vi "SLL DE AI Circular Buffer.vi"(6 "Pointers":T3=enum."Pointer 4", 7 "Options":T4=enum."Write", 8 "error in (no error)":errorcluster, 9 "Time In":timestamp[](array[timestamp]), 11 "Input Data":sgl[][](array[numeric])) -> (0 "error Out":errorcluster, 1 "Data Overflow?":T1, 2 "Output points":sgl[](array[numeric]), 3 "Output Data":sgl[][](array[numeric]), 4 "Multi Time Stamp":timestamp[](array[timestamp]), 5 "Single Time Stamp":timestamp)   [LabVIEW 2009]
doc: "This vi acts as a circular buffer for Analog input channel data storage. \nOutput Array- Column coresponds to single channel data.\nSingle Point data of all channels will avilable, When 'Data Point' case will executes.\nYou can get continous data in two mode 'Read Pointer 1' and 'Read Pointer 2'.\nInitializing Pointer is recommeded to avoid overflow\n\nCreated by Yogesh Redemptor, \nCopyright © 2009, Soliton Technologies.\nAll rights reserved."
uses:
  Controls/SLL DE Circular Buffer Options.ctl
  Controls/SLL DE Circular Buffer Pointers List.ctl
  Controls/SLL DE List of Analog Inputs.ctl
  Controls/SLL DE Circular Buffer Overflow Info.ctl
  Controls/SLL DE DAQ Parameters LV2Global Options.ctl
panel:
  in  "List of Analog Inputs":T2
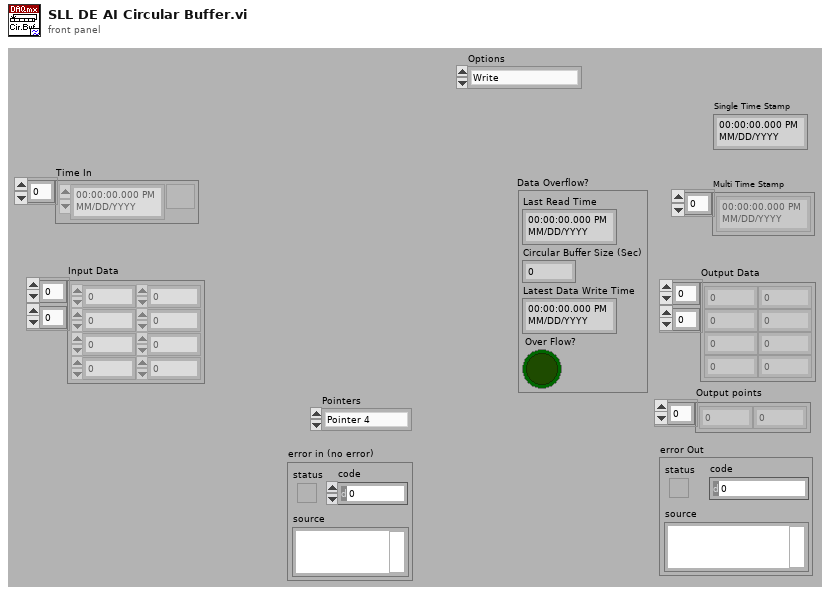
[diagram p1: front panel]
types:
  T1 = typedef "SLL DE Circular Buffer Overflow Info.ctl" = cluster{"Last Read Time":timestamp, "Circular Buffer Size (Sec)":dbl, "Latest Data Write Time":timestamp, "Over Flow?":bool}
  T2 = typedef "SLL DE List of Analog Inputs.ctl" = enum16{"None"}
  T3 = typedef "SLL DE Circular Buffer Pointers List.ctl" = enum16{"Graph Pointer", "File Log Pointer", "Pointer 3", "Pointer 4"}
  T4 = typedef "SLL DE Circular Buffer Options.ctl" = enum16{"Initialize", "Init Pointer X", "Write", "Read Single Value", "Read Pointer X (Multi Value)", "Clear Data"}
  T5 = typedef "SLL DE DAQ Parameters LV2Global Options.ctl" = enum16{"Read", "Write"}
  T6 = cluster{"Buffer Length":i32, "Write Pointer":i32, "Write Time":timestamp}
  T7 = cluster{"Read Pointer X Pointer":i32, "Pointer X Overflow?":bool, "Read Pointer X Time":timestamp}
  T8 = typedef "SLL DE DAQ Engine Parameters.ctl" = cluster{"Enable Engines":cluster{"AI Enable":bool, "AO Enable":bool, "DI Enable":bool, "DO Enable":bool}, "DAQ Control Type":cluster{"Analog Input":enum16{"Finite", "Continuous", "Driver"}, "Analog Output":enum16{"Finite", "Continuous", "Driver"}, "Digital Input":enum16{"Finite", "Continuous", "Driver"}, "Digital Output":enum16{"Finite", "Continuous", "Driver"}}, "DAQ Parameters":cluster{"AI Sampling Rate (Samples/Sec)":dbl, "MvgAVG Window Size (# of Points)":i32, "Enable Filter":bool, "Enable MvgAVG":bool, "Circular Buffer Size (Sec)":dbl, "AO Sampling Rate (Samples/Sec)":dbl, "Graph Update Rate (Samples/Sec)":dbl, "File Logging Rate (Samples/Sec)":i32}, "AO Safe Values":cluster{"Analog Outputs Name":T9, "Analog Outputs Safe Value":dbl}[], "DO Safe Values":cluster{"Digital Outputs Name":T10, "Digital Outputs Safe Value":bool}[], "DO Interconnected Lines":cluster{"First DO Line":string, "Second DO Line":string}[], "AI Channels Unit":cluster{"Channel Name":T2, "Channel Type":T11}[], "Units Information":cluster{"Channel Type":T11, "Unit Text":string, "Maximum":dbl, "Minmum":dbl, "Increments":dbl}[]}
  T9 = typedef "SLL DE List of Analog Outputs.ctl" = enum16{"None"}
  T10 = typedef "SLL DE List of Digital Outputs.ctl" = enum16{"STATION1_START TEST", "STATION1_STOP TEST", "STATION1_LIGHT1", "STATION1_LIGHT2", "STATION1_LIGHT3", "STATION2_START TEST", "STATION2_STOP TEST", "STATION2_LIGHT1", "STATION2_LIGHT2", "STATION2_LIGHT3", "STATION3_START TEST", "STATION3_STOP TEST", "STATION3_LIGHT1", "STATION3_LIGHT2", "STATION3_LIGHT3", "STATION4_START TEST", "STATION4_STOP TEST", "STATION4_LIGHT1", "STATION4_LIGHT2", "STATION4_LIGHT3"}
  T11 = typedef "SLL DE List of AI Channel Type.ctl" = enum16{"Pressure", "Flow", "Temperature", "Time Scale", "Voltage", "Current", "Frequency", "Sound", "Speed", "Torque", "Distance", "Channel Type 1", "Channel Type 2", "Channel Type 3"}
  T12 = cluster{"Read Pointer X Pointer":i32, "Pointer X Overflow?":bool, "Read Pointer X Time":timestamp}[]
  T13 = cluster{"Read Pointer X Time":timestamp, "Circular Buffer Size (Sec)":dbl, "Write Time":timestamp, bool}
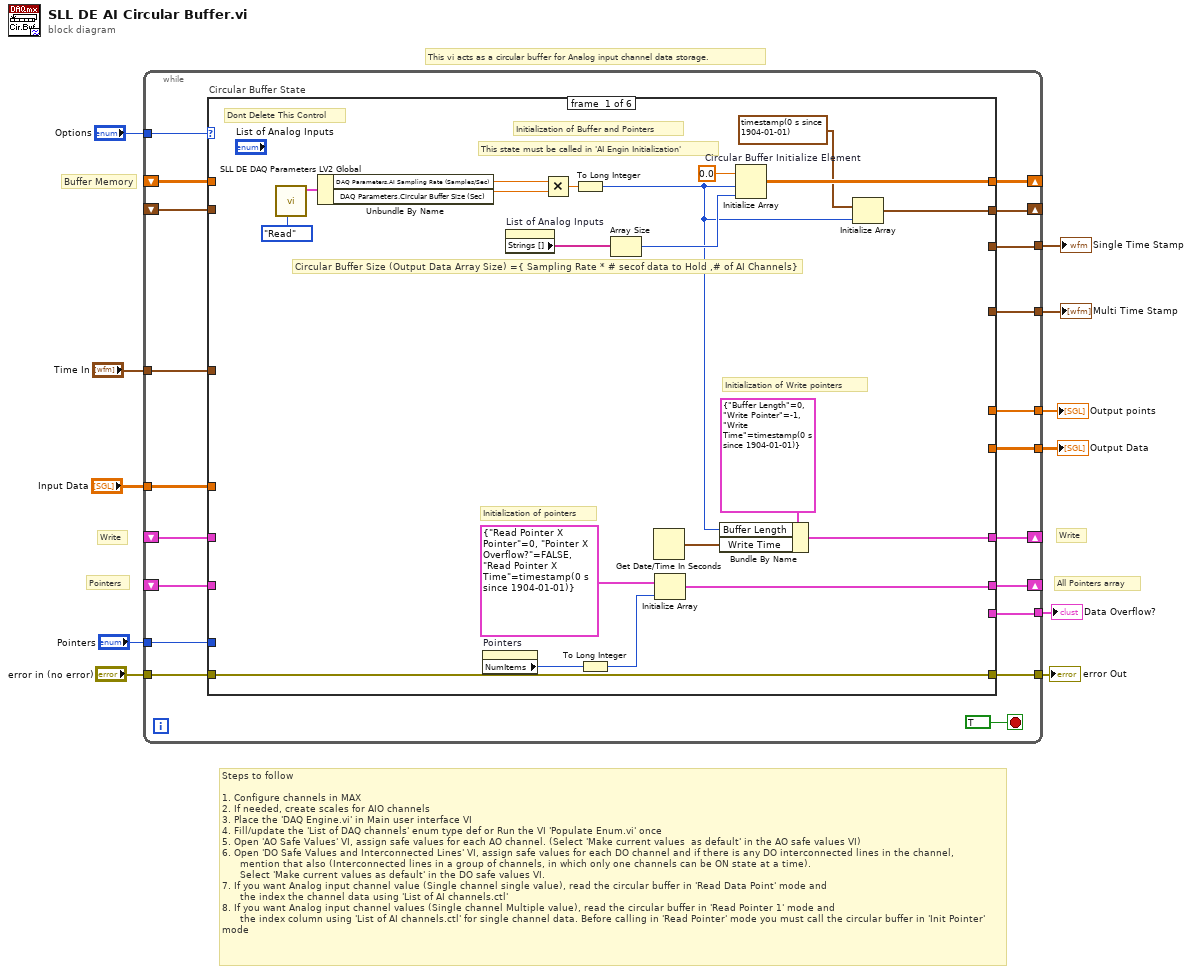
[diagram p0: block diagram]
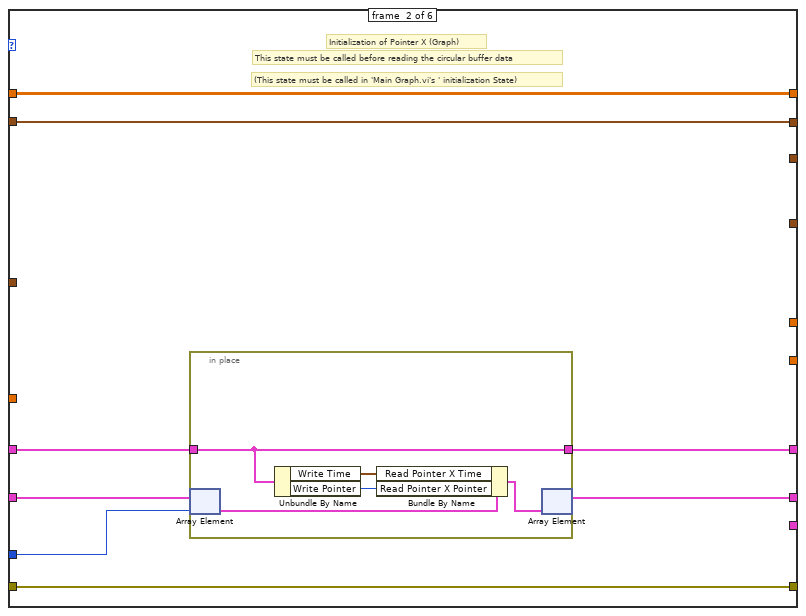
[diagram p2: hidden frame]
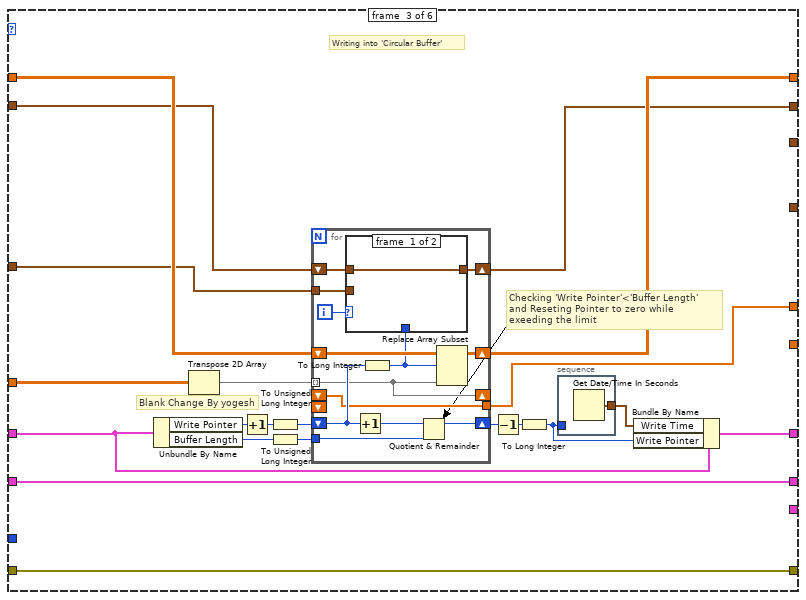
[diagram p3: hidden frame]
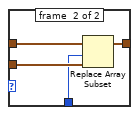
[diagram p4: hidden frame]
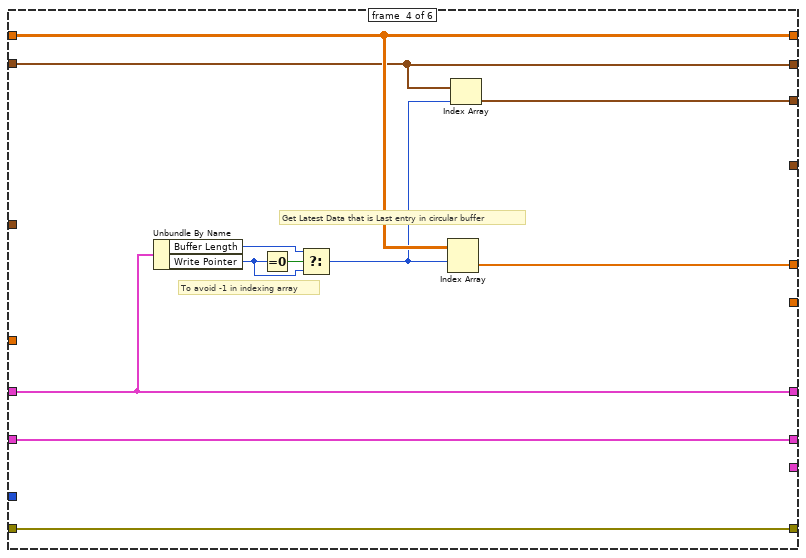
[diagram p5: hidden frame]
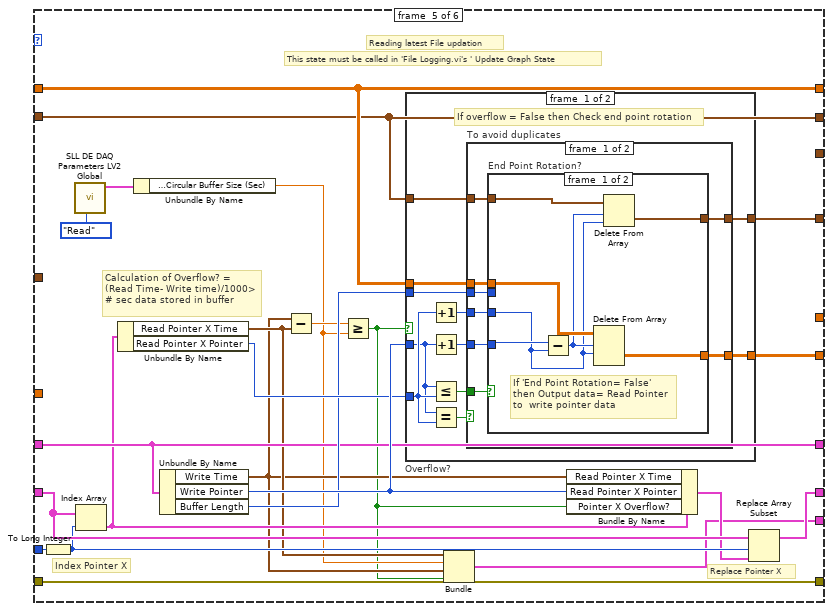
[diagram p6: hidden frame]
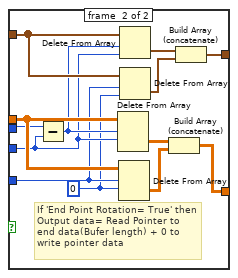
[diagram p7: hidden frame]
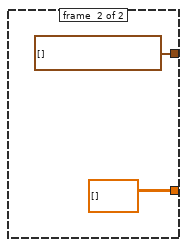
[diagram p8: hidden frame]
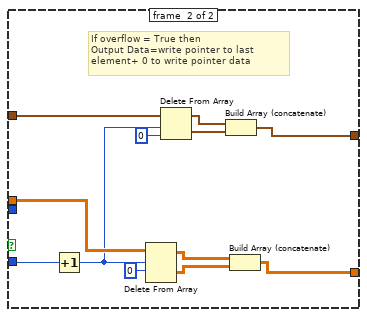
[diagram p9: hidden frame]
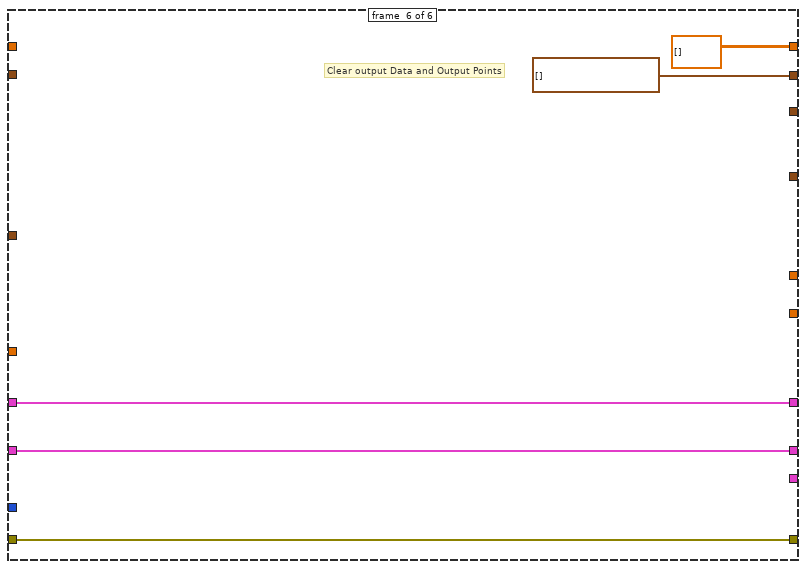
[diagram p10: hidden frame]
diagram:
  # "Steps to follow\n\n1.\tConfigure channels in MAX\n2.\tIf needed, create scales for AIO channels\n3.\tPlace the 'DAQ Engine.vi' in Main user interface VI\n4.\tFill/update the 'List of DAQ channels' enum type def or Run the VI 'Populate Enum.vi' once\n5.\tOpen 'AO Safe Values' VI, assign safe values for each AO channel. (Select 'Make current values  as default' in the AO safe values VI)\n6.\tOpen 'DO Safe Values and Interconnected Lines' VI, assign safe values for each DO channel and if there is any DO interconnected lines in the channel,\n      mention that also (Interconnected lines in a group of channels, in which only one channels can be ON state at a time). \n      Select 'Make current values as default' in the DO safe values VI.\n7.\tIf you want Analog input channel value (Single channel single value), read the circular buffer in 'Read Data Point' mode and \n      the index the channel data using 'List of AI channels.ctl' \n8.\tIf you want Analog input channel values (Single channel Multiple value), read the circular buffer in 'Read Pointer 1' mode and \n      the index column using 'List of AI channels.ctl' for single channel data. Before calling in 'Read Pointer' mode you must call the circular buffer in 'Init Pointer' mode"
  # "Buffer Memory"
  # "Write"
  # "Write"
  # "Pointers"
  # "All Pointers array"
  # "This vi acts as a circular buffer for Analog input channel data storage."
  n1 = while {
    tunnel: "Options" -> [w31]
    shift-right: [w29] -> _
    shift-left: _ -> [w27]
    shift-right: [w28] -> _
    shift-left: _ -> [w26]
    tunnel: "Input Data" -> [w25]
    tunnel: [w24] -> w10
    shift-right: [w23] -> _
    shift-left: _ -> [w22]
    tunnel: [w21] -> w9
    tunnel: "error in (no error)" -> [w20]
    tunnel: [w19] -> w7
    tunnel: "Pointers" -> [w18]
    tunnel: "Time In" -> [w17]
    shift-right: [w16] -> _
    shift-left: _ -> [w15]
    tunnel: [w14] -> w3
    tunnel: [w13] -> w2
    tunnel: [w12] -> w1
    stop <- TRUE stop-if-true
    n2 = case "Circular Buffer State" shown="\"Read Pointer X (Multi Value)\"" w31 {
      tunnel: [w51 w59 w81 w114 w138 sgl[][] []] -> w29
      tunnel: [w46 w55 w85 w115 w127 w196] -> w28
      tunnel: w27 -> [_ w59 w83 w114 w138 _]
      tunnel: w26 -> [_ w57 w85 w115 w130 w196]
      tunnel: w25 -> [_ _ w84 _ _ _]
      tunnel: [_ _ w69 w113 _ _] -> w24
      tunnel: [w47 w54 w82 w112 w133 w195] -> w23
      tunnel: w22 -> [_ w52 w78 w112 w133 w195]
      tunnel: [_ _ _ _ w137 _] -> w21
      tunnel: w20 -> [w36 w58 w70 w108 w132 w193]
      tunnel: [w36 w58 w70 w108 w132 w193] -> w19
      tunnel: w18 -> [_ w56 _ _ w131 _]
      tunnel: w17 -> [_ _ w67 _ _ _]
      tunnel: [w40 w53 w66 w107 w124 timestamp[] []] -> w16
      tunnel: w15 -> [_ w53 w68 w107 w124 _]
      tunnel: [_ _ _ w105 _ _] -> w14
      tunnel: [_ _ _ _ w125 _] -> w13
      tunnel: [_ _ _ _ w116 _] -> w12
      frame #0 {
        w50 = sgl 0.0  # Circular Buffer Initialize Element
        # "Dont Delete This Control"
        # "Initialization of pointers"
        # "Initialization of Write pointers"
        # "This state must be called in 'AI Engin Initialization'"
        # "Initialization of Buffer and Pointers"
        # "Circular Buffer Size (Output Data Array Size) ={ Sampling Rate * # secof data to Hold ,# of AI Channels}"
        n3 = call "SLL DE DAQ Parameters LV2 Global.vi"("Option"=SLL_DE_DAQ_Parameters_LV2Global_Options."Read") -> ("Global Info"=w37:T8)  [unwired: 9 in, 1 out]
        n4 = Unbundle By Name(w37) -> ("DAQ Parameters.AI Sampling Rate (Samples/Sec)"=w39:dbl, "DAQ Parameters.Circular Buffer Size (Sec)"=w33:dbl)
        n5 = property on="Pointers" class="Enum (strict)"() -> ("NumItems"=w35:u32)  [unwired: 2 in, 2 out]
        n6 = property on="List of Analog Inputs" class="Enum (strict)"() -> ("Strings []"=w44:string[])  [unwired: 2 in, 2 out]
        n7 = Multiply(x=w39, y=w33) -> (x*y=w49:dbl)
        n8 = To Long Integer(number=w49) -> (32bit integer=w41:i32)
        n9 = To Long Integer(number=w35) -> (32bit integer=w34:i32)
        n10 = Array Size(array=w44) -> (size(s)=w43:i32)
        n11 = Get Date/Time In Seconds() -> (seconds since 1Jan1904=w32:timestamp)
        n12 = Initialize Array(T7 {"Read Pointer X Pointer"=0, "Pointer X Overflow?"=FALSE, "Read Pointer X Time"=timestamp(0 s since 1904-01-01)} ("Graph"), w34) -> (w46:T12)
        n13 = Bundle By Name(cluster=T6 {"Buffer Length"=0, "Write Pointer"=-1, "Write Time"=timestamp(0 s since 1904-01-01)} ("Cluster"), "Buffer Length"=w41, "Write Time"=w32) -> (w47:T6)
        n14 = Initialize Array(w50, w41, w43) -> (w51:sgl[][])
        n15 = Initialize Array(timestamp(0 s since 1904-01-01), w41) -> (w40:timestamp[])
      }
      frame #1 {
        # "(This state must be called in 'Main Graph.vi's ' initialization State)"
        # "Initialization of Pointer X (Graph)"
        # "This state must be called before reading the circular buffer data"
        n16 = in-place {
          in-place-border: w52 -> [w60]
          in-place-border: [w60] -> w54
          n17 = in-place-array #1(w57, w56) -> (w62:T7)
          n18 = Unbundle By Name(w60) -> ("Write Time"=w64:timestamp, "Write Pointer"=w63:i32)
          n19 = Bundle By Name(cluster=w62, "Read Pointer X Time"=w64, "Read Pointer X Pointer"=w63) -> (w61:T7)
          n20 = in-place-array #1(w61) -> (w55:T12)  [unwired: 1 out]
        }
      }
      frame #2 {
        # "Blank Change By yogesh"
        # "Writing into 'Circular Buffer'"
        # "Checking 'Write Pointer'<'Buffer Length'  and Reseting Pointer to zero while exeeding the limit"
        n21 = Unbundle By Name(w78) -> ("Write Pointer"=w80:i32, "Buffer Length"=w79:i32)
        n22 = Transpose 2D Array(2D array=w84) -> (transposed array=w74:sgl[][])
        n23 = Increment(x=w80) -> (x+1=w71:i32)
        n24 = To Unsigned Long Integer(number=w71) -> (unsigned 32bit integer=w76:u32)
        n25 = To Unsigned Long Integer(number=w79) -> (unsigned 32bit integer=w75:u32)
        n26 = for {
          tunnel: w74 -> [w93] mode=indexing
          shift-right: [w96] -> w77
          shift-left: w76 -> [w95]
          shift-right: [w98] -> w81
          shift-left: w83 -> [w99]
          tunnel: w75 -> [w97]
          shift-right: [w93] -> _
          shift-left: _ -> [w92]
          shift-left: _ -> [_]
          tunnel: [w92] -> w69
          shift-right: [w90] -> w66
          shift-left: w68 -> [w91]
          tunnel: w67 -> [w89]
          i -> [w87]
          n27 = Increment(x=w95) -> (x+1=w94:u32)
          n28 = To Long Integer(number=w95) -> (32bit integer=w88:i32)
          n29 = case shown="0" w87 {
            tunnel: w91 -> [w100 w104]
            tunnel: [w100 w103] -> w90
            tunnel: w89 -> [_ w102]
            tunnel: w88 -> [_ w101]
            frame #0 {
            }
            frame #1 {
              n30 = Replace Array Subset(array=w104, new element=w102, index=w101) -> (w103:timestamp[])
            }
          }
          n31 = Quotient & Remainder(x=w94, y=w97) -> (x-y*floor(x/y)=w96:u32)  [unwired: 1 out]
          n32 = Replace Array Subset(array=w99, new element=w93, index (row)=w88) -> (w98:sgl[][])  [unwired: 1 in]
        }
        n33 = Decrement(x=w77) -> (x-1=w72:u32)
        n34 = To Long Integer(number=w72) -> (32bit integer=w65:i32)
        n35 = stacked-sequence {
          tunnel: [w86] -> w73
          tunnel: w65 -> [_]
          frame #0 {
            n36 = Get Date/Time In Seconds() -> (seconds since 1Jan1904=w86:timestamp)
          }
        }
        n37 = Bundle By Name(cluster=w78, "Write Time"=w73, "Write Pointer"=w65) -> (w82:T6)
      }
      frame #3 {
        # "To avoid -1 in indexing array"
        # "Get Latest Data that is Last entry in circular buffer"
        n38 = Unbundle By Name(w112) -> ("Buffer Length"=w110:i32, "Write Pointer"=w109:i32)
        n39 = Equal To 0?(x=w109) -> (x = 0?=w111:bool)
        n40 = Select(t=w110, s=w111, f=w109) -> (s? t:f=w106:i32)
        n41 = Index Array(array=w114, index (row)=w106) -> (element=w113:sgl[])  [unwired: 1 in]
        n42 = Index Array(array=w107, index=w106) -> (element=w105:timestamp)
      }
      frame #4 {
        # "Replace Pointer X"
        # "Index Pointer X"
        # "Calculation of Overflow? = \n(Read Time- Write time)/1000> # sec data stored in buffer"
        # "Reading latest File updation"
        # "This state must be called in 'File Logging.vi's ' Update Graph State"
        n43 = To Long Integer(number=w131) -> (32bit integer=w129:i32)
        n44 = call "SLL DE DAQ Parameters LV2 Global.vi"("Option"=SLL_DE_DAQ_Parameters_LV2Global_Options."Read") -> ("Global Info"=w123:T8)  [unwired: 9 in, 1 out]
        n45 = Index Array(array=w130, index=w129) -> (element=w126:T7)
        n46 = Unbundle By Name(w126) -> ("Read Pointer X Time"=w120:timestamp, "Read Pointer X Pointer"=w135:i32)
        n47 = Unbundle By Name(w123) -> ("DAQ Parameters.Circular Buffer Size (Sec)"=w118:dbl)
        n48 = Unbundle By Name(w133) -> ("Write Time"=w119:timestamp, "Write Pointer"=w136:i32, "Buffer Length"=w134:i32)
        n49 = Subtract(x=w119, y=w120) -> (x-y=w121:dbl)
        n50 = Greater Or Equal?(x=w121, y=w118) -> (x >= y?=w117:bool)
        n51 = case "Overflow?" shown="False" w117 {
          tunnel: w138 -> [w148 w189]
          tunnel: [w147 w187] -> w137
          tunnel: w136 -> [w143 w191]
          tunnel: w135 -> [w144 _]
          tunnel: w134 -> [w146 _]
          tunnel: w124 -> [w140 w185]
          tunnel: [w139 w180] -> w125
          frame #0 {
            # "If overflow = False then Check end point rotation"
            n52 = Increment(x=w144) -> (x+1=w141:i32)
            n53 = Increment(x=w143) -> (x+1=w142:i32)
            n54 = Less Or Equal?(x=w143, y=w144) -> (x <= y?=w149:bool)
            n55 = Equal?(x=w143, y=w144) -> (x = y?=w145:bool)
            n56 = case "To avoid duplicates" shown="False" w145 {
              tunnel: w149 -> [w157 _]
              tunnel: w148 -> [w156 _]
              tunnel: [w155 sgl[][] []] -> w147
              tunnel: w146 -> [w154 _]
              tunnel: w141 -> [w153 _]
              tunnel: w142 -> [w152 _]
              tunnel: w140 -> [w151 _]
              tunnel: [w150 timestamp[] []] -> w139
              frame #0 {
                n57 = case "End Point Rotation?" shown="False" w157 {
                  tunnel: w156 -> [w164 w177]
                  tunnel: [w163 w174] -> w155
                  tunnel: w153 -> [w159 w170]
                  tunnel: w152 -> [w162 w169]
                  tunnel: w154 -> [_ w173]
                  tunnel: w151 -> [w161 w172]
                  tunnel: [w158 w165] -> w150
                  frame #0 {
                    # "If 'End Point Rotation= False' then Output data= Read Pointer to  write pointer data"
                    n58 = Subtract(x=w162, y=w159) -> (x-y=w160:i32)
                    n59 = Delete From Array(array=w164, length=w160, index (row)=w159) -> (deleted portion=w163:sgl[][])  [unwired: 1 in, 1 out]
                    n60 = Delete From Array(array=w161, length=w160, index=w159) -> (deleted portion=w158:timestamp[])  [unwired: 1 out]
                  }
                  frame #1 {
                    w168 = 0 ("index (row)")
                    # "If 'End Point Rotation= True' then Output data= Read Pointer to end data(Bufer length) + 0 to write pointer data"
                    n61 = Subtract(x=w173, y=w170) -> (x-y=w171:i32)
                    n62 = Delete From Array(array=w177, length=w171, index (row)=w170) -> (deleted portion=w176:sgl[][])  [unwired: 1 in, 1 out]
                    n63 = Delete From Array(array=w177, length=w169, index (row)=w168) -> (deleted portion=w175:sgl[][])  [unwired: 1 in, 1 out]
                    n64 = Delete From Array(array=w172, length=w171, index=w170) -> (deleted portion=w166:timestamp[])  [unwired: 1 out]
                    n65 = Delete From Array(array=w172, length=w169, index=w168) -> (deleted portion=w167:timestamp[])  [unwired: 1 out]
                    n66 = Build Array (concatenate)(w176, w175) -> (w174:sgl[][])
                    n67 = Build Array (concatenate)(w166, w167) -> (w165:timestamp[])
                  }
                }
              }
              frame #1 {
              }
            }
          }
          frame #1 {
            # "If overflow = True then\nOutput Data=write pointer to last element+ 0 to write pointer data"
            n68 = Increment(x=w191) -> (x+1=w184:i32)
            n69 = Delete From Array(array=w189, length=w184, index (row)=0) -> (deleted portion=w188:sgl[][], array with subset deleted=w186:sgl[][])  [unwired: 1 in]
            n70 = Delete From Array(array=w185, length=w184, index=0 ("index (row)")) -> (deleted portion=w181:timestamp[], array with subset deleted=w182:timestamp[])
            n71 = Build Array (concatenate)(w182, w181) -> (w180:timestamp[])
            n72 = Build Array (concatenate)(w186, w188) -> (w187:sgl[][])
          }
        }
        n73 = Bundle("Read Pointer X Time"=w120, "Circular Buffer Size (Sec)"=w118, "Write Time"=w119, w117) -> (w116:T13)  [unwired: 1 in]
        n74 = Bundle By Name(cluster=w126, "Read Pointer X Time"=w119, "Read Pointer X Pointer"=w136, "Pointer X Overflow?"=w117) -> (w128:T7)
        n75 = Replace Array Subset(array=w130, new element=w128, index=w129) -> (w127:T12)
      }
      frame #5 {
        # "Clear output Data and Output Points"
      }
    }
  }
  "Output Data" <- w9
  "Output points" <- w10
  "error Out" <- w7
  "Single Time Stamp" <- w3
  "Multi Time Stamp" <- w2
  "Data Overflow?" <- w1
